vi "Upgrade dotNET Socket to SSL.vi"(8 "error in (no error)":errorcluster, 10 "Hostname / URL":string="echo.websocket.org:443", 11 "dotNET TCP Socket in":refnum<class "dotNET TCP Socket.lvclass">) -> (0 "error out":errorcluster, 3 "dotNET SSL Client Socket out":refnum<class "dotNET SSL Client Socket.lvclass">)   [LabVIEW 2013, in "dotNET SSL Socket.lvlib" / "dotNET SSL Client Socket.lvclass"]
doc: "Upgrades a dotNET TCP Socket object to an SSL Client Socket. After calling this VI, the SSL options should be set and then the Handshake VI called."
uses:
  dotNET SSL Client Socket.lvclass
  dotNET TCP Socket/dotNET TCP Socket.lvclass
  dotNET TCP Socket/dotNET TCP Socket.lvclass/dotNET TCP Socket.ctl
  Z:/LabVIEW Working Directory/MediaMongrels Library Packages/secure-websockets-addon/Source/dotNET SSL Socket/TimeoutSSLStream.dll
  TimeoutSSLStream.dll
  dotNET SSL Socket/dotNET SSL Socket.lvclass/dotNET SSL Socket.ctl
  dotNET SSL Client Socket.lvclass/dotNET SSL Client Socket.ctl
  dotNET TCP Socket/Read TcpClient.vi
  dotNET SSL Socket/Write SSLStream.vi
  Write Hostname _ URL.vi
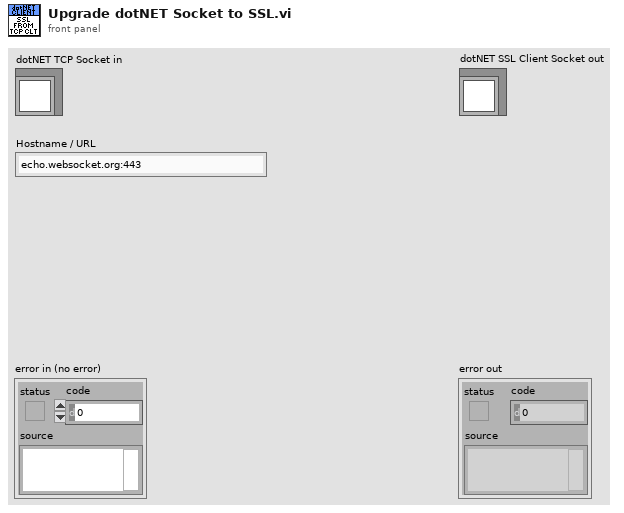
[diagram p1: front panel]
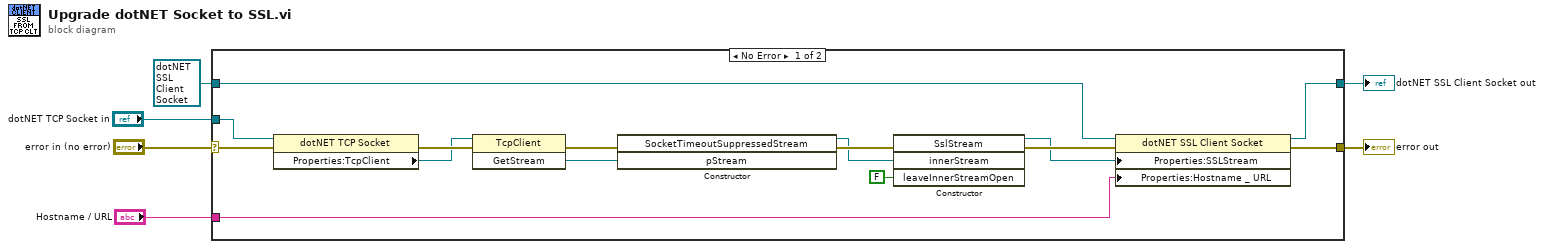
[diagram p0: block diagram]
diagram:
  n1 = case shown="No Error" "error in (no error)" {
    selector: "error in (no error)" -> [w20 w23]
    tunnel: [w16 w23] -> w5
    tunnel: [w17 w22] -> w4
    tunnel: "dotNET TCP Socket in" -> [w12 _]
    tunnel: refnum<class "dotNET SSL Client Socket.lvclass"> refnum ("dotNET SSL Client Socket in") -> [w15 w22]
    tunnel: "Hostname / URL" -> [w14 _]
    frame No Error {
      n2 = property class="dotNET TCP Socket"(reference=w12, error in=w20) -> (error out=w13:errorcluster, "Properties:TcpClient"=w11:refnum<k24>)  [unwired: 1 out]
      n3 = invoke class="TcpClient" method="GetStream"(reference=w11, error in=w13) -> (error out=w10:errorcluster, "GetStream"=w9:refnum<k24>)  [unwired: 1 in, 1 out]
      n4 = constructor class="SocketTimeoutSuppressedStream"(error in=w10, "pStream"=w9) -> (reference out=w7:refnum<k24>, error out=w8:errorcluster)  [unwired: 2 in, 2 out]
      n5 = constructor class="SslStream"(error in=w8, "innerStream"=w7, "leaveInnerStreamOpen"=FALSE) -> (reference out=w18:refnum<k24>, error out=w19:errorcluster)  [unwired: 2 in, 3 out]
      n6 = property class="dotNET SSL Client Socket"(reference=w15, error in=w19, "Properties:SSLStream"=w18, "Properties:Hostname _ URL"=w14) -> (reference out=w17:refnum<class "dotNET SSL Client Socket.lvclass">, error out=w16:errorcluster)
    }
    frame Error {
    }
  }
  "error out" <- w5
  "dotNET SSL Client Socket out" <- w4
